vi "Get Public API.vi"(8 "error in (no error)":errorcluster, 11 "instrument.PPMS2 in":refnum<class "instrument.PPMS.lvclass">) -> (0 "error out":errorcluster, 2 "Commands":string[](array[string]), 3 "instrument.PPMS2 out":refnum<class "instrument.PPMS.lvclass">)   [LabVIEW 2016, in "instrument.PPMS.lvclass"]
uses:
  instrument.PPMS.lvclass
  <userlib>/LevyLab/Levylab Instruments/Instrument Types/Cryostat/Instrument.Cryostat.lvclass
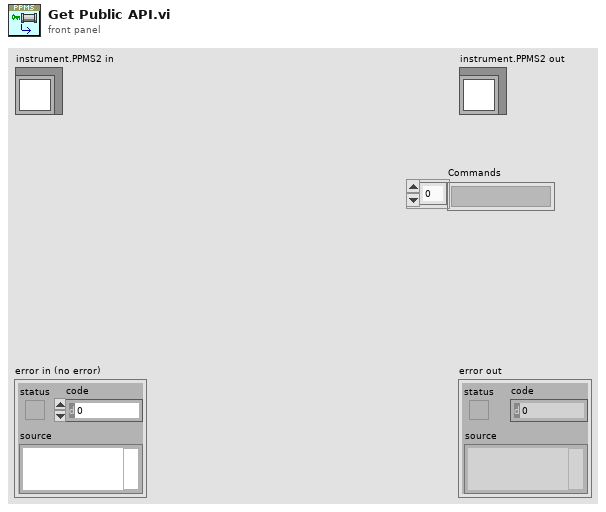
[diagram p1: front panel]
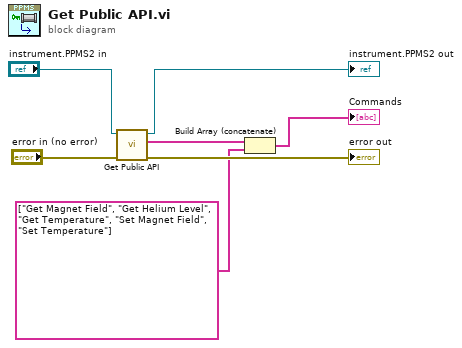
[diagram p0: block diagram]
diagram:
  n1 = call-parent "Get Public API.vi"("error in (no error)"="error in (no error)", "Instrument in"="instrument.PPMS2 in") -> ("error out"=→"error out":errorcluster, "Commands"=w1:string[], "Instrument out"=→"instrument.PPMS2 out":refnum<class "instrument.PPMS.lvclass">)  [unwired: 7 in]
  n2 = Build Array (concatenate)(w1, string[] ["Get Magnet Field", "Get Helium Level", "Get Temperature", "Set Magnet Field", "Set Temperature"] ("Commands")) -> (→"Commands":string[])
